vi "Main Page.vi"(8 "error in (no error)":errorcluster, 11 "Node Ptr":T1 format="%.0x") -> (0 "error out":errorcluster)   [LabVIEW 2026, in "WebPage Addon System Explorer.lvlib"]
uses:
  WebPage Addon System Explorer.lvlib
  <vilib>/NI VeriStand/Custom Device API/Custom Device Item Ref.ctl
  Types/Main.Settings.ctl
  Types/Page Settings Action.ctl
  <vilib>/NI VeriStand/Custom Device API/Custom Device API.lvlib
  Addon Shared/Constants.vi
  Addon Shared/WebPage Addon Shared.lvlib
panel:
  out "gRPC Address":string
  out "Webpage Address":string
  in  "gRPC Port":u32=53251
  in  "Hosted Port":u32=8382
  in  "Hosted IP Address":string
  out "Published Channels":string[][](table)
  in  "Update Rate (Hz)":dbl=1.0 min=0.5 max=100.0 step=0.5
  out "Version":string
  in  "SHDocVw.IWebBrowser":refnum<k7>(container)
  in  "Specific Header":cluster{"Section Name":string}={"Section Name"="Custom Device Item Settings"}
  in  "General Header":cluster{"Section Name":string}={"Section Name"="General Custom Device Settings"}
  in  "Name":string
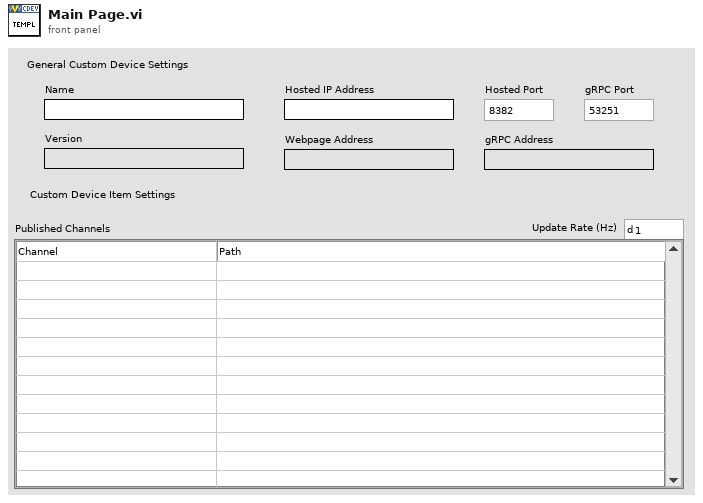
[diagram p1: front panel]
types:
  T1 = typedef "Custom Device API.lvlib/Custom Device Item Ref.ctl" = u64
  T2 = typedef "WebPage Addon System Explorer.lvlib/Page Settings Action.ctl" = enum16{"Get", "Set"}
  T3 = typedef "WebPage Addon System Explorer.lvlib/Main.Settings.ctl" = cluster{"Update Rate":dbl, "Hosted Port":u32, "gRPC Port":u32, "Hosted IP Address":string}
  T4 = typedef "Custom Device API.lvlib/Custom Device Item Info.ctl" = cluster{"Name":string, "Is Channel":bool, "GUID":string, "Is Waveform":bool}
  T5 = typedef "Custom Device API.lvlib/Custom Device Pointer.ctl" = refnum<k24>
  T6 = typedef "Custom Device API.lvlib/Custom Device Commands.ctl" = enum16{"Default", "Item renamed", "Shutdown", "Dynamic button pressed"}
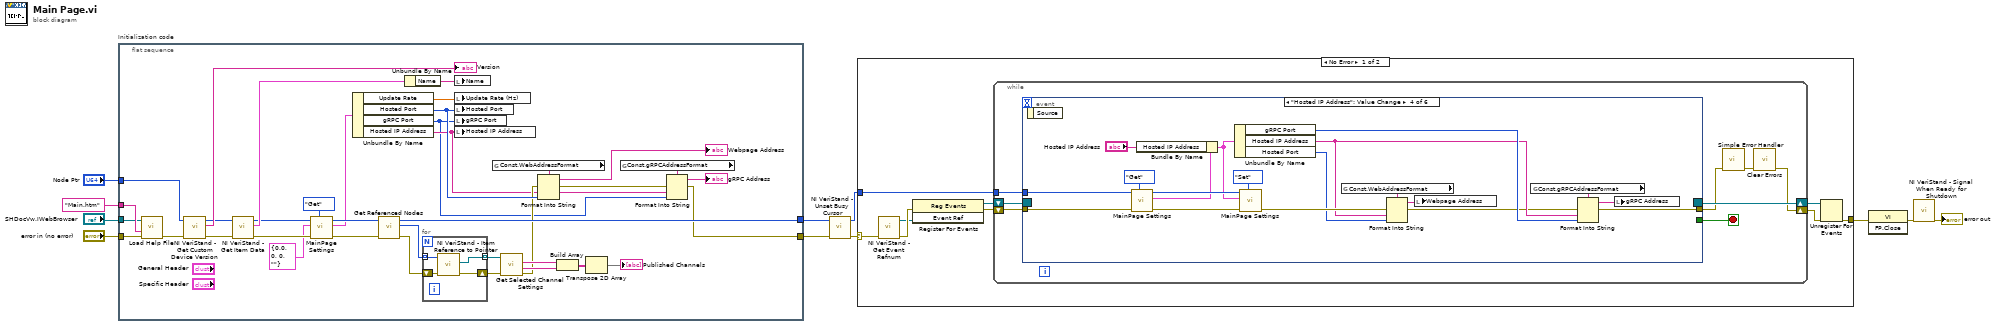
[diagram p0: block diagram]
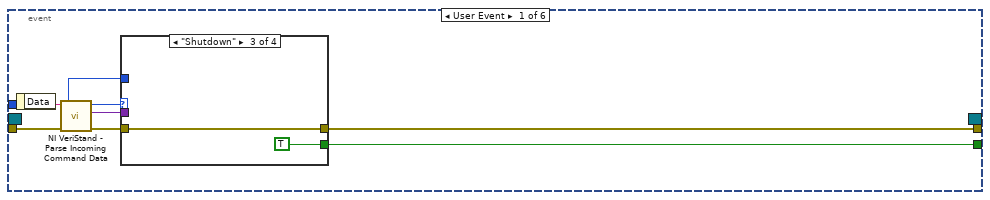
[diagram p2: hidden frame]
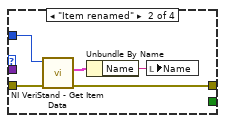
[diagram p4: hidden frame]
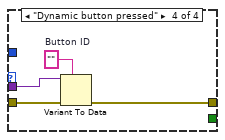
[diagram p5: hidden frame]
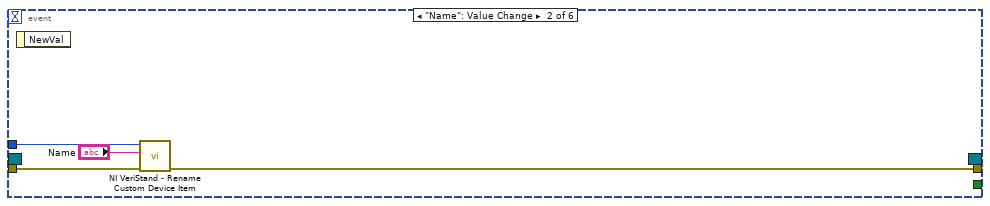
[diagram p6: hidden frame]
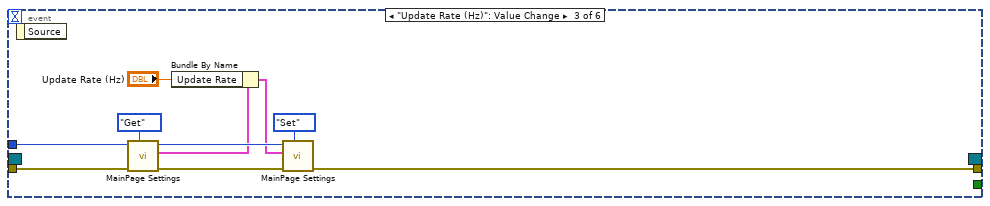
[diagram p7: hidden frame]
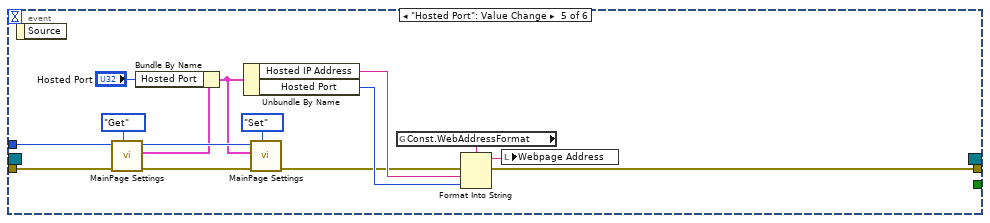
[diagram p8: hidden frame]
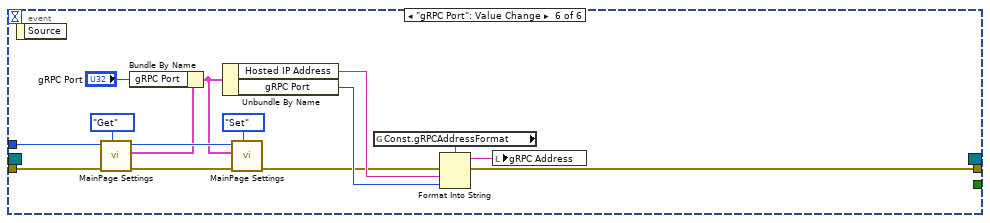
[diagram p9: hidden frame]
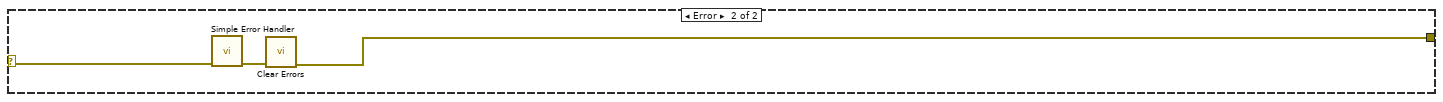
[diagram p10: hidden frame]
diagram:
  n1 = flat-sequence "Initialization code" {
    tunnel: "error in (no error)" -> [w43]
    tunnel: "Node Ptr" -> [w46]
    tunnel: [w16] -> w6
    tunnel: [w37] -> w3
    tunnel: "SHDocVw.IWebBrowser" -> [w40]
    tunnel: "Main.htm" ("HTML File") -> [w41]
    frame #0 {
      n2 = call "Load Help File.vi"("error in (no error)"=w43, "HTML File to Load"=w41, "Browser"=w40) -> ("error out"=w42:errorcluster)  [unwired: 8 in]
      n3 = call <vilib>:"NI VeriStand - Get Custom Device Version.vi"("error in (no error)"=w42, "Device Ref in"=w46) -> ("error out"=w28:errorcluster, "Value"=→"Version":string, "Device Ref out"=w27:T1)  [unwired: 7 in]
      n4 = call <vilib>:"NI VeriStand - Get Item Data.vi"("error in (no error)"=w28, "Item Ref in"=w27) -> ("error out"=w39:errorcluster, "Item Info"=w47:T4, "Item Ref out"=w38:T1)  [unwired: 7 out]
      n5 = call "MainPage Settings.vi"("Action"=Page_Settings_Action."Get", "error in (no error)"=w39, "Settings In"=T3 {"Update Rate"=0.0, "Hosted Port"=0, "gRPC Port"=0, "Hosted IP Address"=""} ("cluster"), "Item Ref in"=w38) -> ("error out"=w26:errorcluster, "Settings Out"=w23:T3, "Item Ref out"=w25:T1)  [unwired: 5 in]
      n6 = Unbundle By Name(w23) -> ("Update Rate"=w22:dbl, "Hosted Port"=w20:u32, "gRPC Port"=w14:u32, "Hosted IP Address"=w15:string)
      n7 = call "Get Referenced Nodes.vi"("error in (no error)"=w26, "Item Ref in"=w25) -> ("error out"=w36:errorcluster, "Array"=w34:T1[], "Item Ref out"=w37:T1)  [unwired: 7 in]
      n8 = Unbundle By Name(w47) -> ("Name"=w44:string)
      n9 = for {
        shift-right: [w50] -> w35
        shift-left: w36 -> [w51]
        tunnel: w34 -> [w49] mode=indexing
        tunnel: [w48] -> w33 mode=indexing
        n10 = call <vilib>:"NI VeriStand - Item Reference to Pointer.vi"("error in (no error)"=w51, "Item Ref in"=w49) -> ("error out"=w50:errorcluster, "Node Pointer"=w48:T5)  [unwired: 6 in, 2 out]
      }
      n11 = local write "Name"(w44) -> ()
      n12 = local write "Update Rate (Hz)"(w22) -> ()
      n13 = local write "Hosted Port"(w20) -> ()
      n14 = local write "gRPC Port"(w14) -> ()
      n15 = local write "Hosted IP Address"(w15) -> ()
      n16 = global read "Constants.vi" "Const.WebAddressFormat"() -> (w12:string)
      n17 = call "Get Selected Channel Settings.vi"("error in (no error)"=w35, "Refs"=w33) -> ("error out"=w17:errorcluster, "Path"=w31:string[], "Name"=w32:string[])  [unwired: 6 in, 1 out]
      n18 = Format Into String(format string=w12, error in=w17, w15, w20) -> (resulting string=→"Webpage Address":string, error out=w18:errorcluster)  [unwired: 1 in]
      n19 = Build Array(w32, w31) -> (w30:string[][])
      n20 = Transpose 2D Array(2D array=w30) -> (transposed array=→"Published Channels":string[][])
      n21 = global read "Constants.vi" "Const.gRPCAddressFormat"() -> (w11:string)
      n22 = Format Into String(format string=w11, error in=w18, w15, w14) -> (resulting string=→"gRPC Address":string, error out=w16:errorcluster)  [unwired: 1 in]
    }
  }
  n23 = call <vilib>:"NI VeriStand - Unset Busy Cursor.vi"("error in (no error)"=w6) -> ("error out"=w5:errorcluster)  [unwired: 10 out]
  n24 = case shown="No Error" w5 {
    selector: w5 -> [w52 w154]
    tunnel: [w57 w152] -> w10
    tunnel: w3 -> [w53 _]
    frame No Error {
      n25 = call <vilib>:"NI VeriStand - Get Event Refnum.vi"("error in (no error)"=w52) -> ("error out"=w60:errorcluster, "Event Ref"=w56:refnum<user-event>)  [unwired: 9 out]
      n26 = register-events(error in=w60, w56) -> (reference out=w54:refnum<event-registration>, error out=w55:errorcluster)  [unwired: 1 in]
      n27 = while {
        tunnel: w53 -> [w64]
        shift-right: [w61] -> w58
        shift-left: w55 -> [w67]
        shift-right: [w68] -> w59
        shift-left: w54 -> [w66]
        stop <- w65 stop-if-true
        n28 = event shown="[3] \"Hosted IP Address\": Value Change" {
          selector: w66 -> [_ _ _ _ _ _]
          dyn-events: [_ _ _ _ _ _] -> w68
          timeout: _ -> [_ _ _ _ _ _]
          tunnel: w67 -> [w76 w92 w97 w116 w131 w145]
          tunnel: [w72 _ _ _ _ _] -> w65
          tunnel: [w71 w91 w96 w103 w122 w138] -> w63
          tunnel: w64 -> [w70 w90 w98 w115 w130 w144]
          event User Event {
            n29 = event-data() -> ("Data"=w75:string)  [unwired: 1 out]
            n30 = call <vilib>:"NI VeriStand - Parse Incoming Command Data.vi"("error in (no error)"=w76, "Incoming data"=w75) -> ("error out"=w74:errorcluster, "Outgoing data"=w69:variant, "Action"=w73:T6)  [unwired: 7 out]
            n31 = case shown="\"Shutdown\"" w73 {
              tunnel: w74 -> [w77 w82 w83 w88]
              tunnel: [_ _ TRUE _] -> w72
              tunnel: [w77 w79 w83 w85] -> w71
              tunnel: w70 -> [_ w81 _ _]
              tunnel: w69 -> [_ _ _ w87]
              frame "Default", Default {
              }
              frame "Item renamed" {
                n32 = call <vilib>:"NI VeriStand - Get Item Data.vi"("error in (no error)"=w82, "Item Ref in"=w81) -> ("error out"=w79:errorcluster, "Item Info"=w80:T4)  [unwired: 8 out]
                n33 = Unbundle By Name(w80) -> ("Name"=w78:string)
                n34 = local write "Name"(w78) -> ()
              }
              frame "Shutdown" {
              }
              frame "Dynamic button pressed" {
                w86 = ""  # Button ID
                n35 = Variant To Data(error in=w88, type=w86, Variant=w87) -> (error out=w85:errorcluster)  [unwired: 1 out]
              }
            }
          }
          event "Name": Value Change {
            n36 = event-data() -> ()  [unwired: 2 out]
            n37 = call <vilib>:"NI VeriStand - Rename Custom Device Item.vi"("error in (no error)"=w92, "New Name"="Name", "Item Ref in"=w90) -> ("error out"=w91:errorcluster)  [unwired: 1 in, 7 out]
          }
          event "Update Rate (Hz)": Value Change {
            n38 = event-data() -> ()  [unwired: 2 out]
            n39 = call "MainPage Settings.vi"("Action"=Page_Settings_Action."Get", "error in (no error)"=w97, "Item Ref in"=w98) -> ("error out"=w100:errorcluster, "Settings Out"=w95:T3, "Item Ref out"=w99:T1)  [unwired: 6 in]
            n40 = Bundle By Name(cluster=w95, "Update Rate"="Update Rate (Hz)") -> (w94:T3)
            n41 = call "MainPage Settings.vi"("Action"=Page_Settings_Action."Set", "error in (no error)"=w100, "Settings In"=w94, "Item Ref in"=w99) -> ("error out"=w96:errorcluster)  [unwired: 5 in, 2 out]
          }
          event "Hosted IP Address": Value Change {
            n42 = event-data() -> ()  [unwired: 2 out]
            n43 = call "MainPage Settings.vi"("Action"=Page_Settings_Action."Get", "error in (no error)"=w116, "Item Ref in"=w115) -> ("error out"=w119:errorcluster, "Settings Out"=w117:T3, "Item Ref out"=w118:T1)  [unwired: 6 in]
            n44 = Bundle By Name(cluster=w117, "Hosted IP Address"="Hosted IP Address") -> (w110:T3)
            n45 = Unbundle By Name(w110) -> ("gRPC Port"=w106:u32, "Hosted IP Address"=w105:string, "Hosted Port"=w109:u32)
            n46 = call "MainPage Settings.vi"("Action"=Page_Settings_Action."Set", "error in (no error)"=w119, "Settings In"=w110, "Item Ref in"=w118) -> ("error out"=w112:errorcluster)  [unwired: 5 in, 2 out]
            n47 = global read "Constants.vi" "Const.WebAddressFormat"() -> (w113:string)
            n48 = Format Into String(format string=w113, error in=w112, w105, w109) -> (resulting string=w111:string, error out=w104:errorcluster)  [unwired: 1 in]
            n49 = local write "Webpage Address"(w111) -> ()
            n50 = global read "Constants.vi" "Const.gRPCAddressFormat"() -> (w108:string)
            n51 = Format Into String(format string=w108, error in=w104, w105, w106) -> (resulting string=w107:string, error out=w103:errorcluster)  [unwired: 1 in]
            n52 = local write "gRPC Address"(w107) -> ()
          }
          event "Hosted Port": Value Change {
            n53 = event-data() -> ()  [unwired: 2 out]
            n54 = call "MainPage Settings.vi"("Action"=Page_Settings_Action."Get", "error in (no error)"=w131, "Item Ref in"=w130) -> ("error out"=w134:errorcluster, "Settings Out"=w132:T3, "Item Ref out"=w133:T1)  [unwired: 6 in]
            n55 = Bundle By Name(cluster=w132, "Hosted Port"="Hosted Port") -> (w124:T3)
            n56 = Unbundle By Name(w124) -> ("Hosted IP Address"=w125:string, "Hosted Port"=w126:u32)
            n57 = call "MainPage Settings.vi"("Action"=Page_Settings_Action."Set", "error in (no error)"=w134, "Settings In"=w124, "Item Ref in"=w133) -> ("error out"=w123:errorcluster)  [unwired: 5 in, 2 out]
            n58 = global read "Constants.vi" "Const.WebAddressFormat"() -> (w128:string)
            n59 = Format Into String(format string=w128, error in=w123, w125, w126) -> (resulting string=w127:string, error out=w122:errorcluster)  [unwired: 1 in]
            n60 = local write "Webpage Address"(w127) -> ()
          }
          event "gRPC Port": Value Change {
            n61 = event-data() -> ()  [unwired: 2 out]
            n62 = call "MainPage Settings.vi"("Action"=Page_Settings_Action."Get", "error in (no error)"=w145, "Item Ref in"=w144) -> ("error out"=w149:errorcluster, "Settings Out"=w147:T3, "Item Ref out"=w148:T1)  [unwired: 6 in]
            n63 = Bundle By Name(cluster=w147, "gRPC Port"="gRPC Port") -> (w137:T3)
            n64 = Unbundle By Name(w137) -> ("Hosted IP Address"=w140:string, "gRPC Port"=w141:u32)
            n65 = call "MainPage Settings.vi"("Action"=Page_Settings_Action."Set", "error in (no error)"=w149, "Settings In"=w137, "Item Ref in"=w148) -> ("error out"=w139:errorcluster)  [unwired: 5 in, 2 out]
            n66 = global read "Constants.vi" "Const.gRPCAddressFormat"() -> (w143:string)
            n67 = Format Into String(format string=w143, error in=w139, w140, w141) -> (resulting string=w142:string, error out=w138:errorcluster)  [unwired: 1 in]
            n68 = local write "gRPC Address"(w142) -> ()
          }
        }
        n69 = call <vilib>:"Simple Error Handler.vi"("error in (no error)"=w63) -> ("error out"=w62:errorcluster)  [unwired: 1 in, 7 out]
        n70 = call <vilib>:"Clear Errors.vi"("error in (no error)"=w62) -> ("error out"=w61:errorcluster)  [unwired: 1 in, 5 out]
      }
      n71 = Unregister For Events(event registration refnum=w59, error in=w58) -> (error out=w57:errorcluster)
    }
    frame Error {
      n72 = call <vilib>:"Simple Error Handler.vi"("error in (no error)"=w154) -> ("error out"=w153:errorcluster)  [unwired: 1 in, 7 out]
      n73 = call <vilib>:"Clear Errors.vi"("error in (no error)"=w153) -> ("error out"=w152:errorcluster)  [unwired: 1 in, 5 out]
    }
  }
  n74 = invoke class="VI" method="FP.Close"(error in=w10) -> (error out=w9:errorcluster)  [unwired: 2 in, 2 out]
  n75 = call <vilib>:"NI VeriStand - Signal When Ready for Shutdown.vi"("error in (no error)"=w9) -> ("error out"=→"error out":errorcluster)  [unwired: 10 out]
